vi "TMC module control_noVISA.vi"(8 "Winkel [°]":dbl min=-360.0 max=360.0 step=0.1, 9 "Nur Position auslesen":bool=TRUE, 10 "error in (no error)":errorcluster, 11 "VISA resource name":refnum<visa-resource-name>="COM6") -> (0 "Ausgelesener Winkel [°]":dbl format="%.1f", 1 "Fehler":bool, 2 "error out":errorcluster, 3 "VISA resource name out":refnum<visa-resource-name>)   [LabVIEW 2019]
doc: "Diese VI steuert einen Steppermotor mit TMCM-110 Modul.\nBei Start laufen folgende Schritte ab:\n1. Wenn \"nur Position auslesen\" deaktiviert ist\n- Überprüfe, ob neu gestartet wurde\n- falls ja: korregiere aktuelle Position auf letze Positionskoordinate vor Abschaltung\n- sende anzufahrende Position (Motor setzt sich in Bewegung)\n- Speichere neue Positions-Koordinate\n- lese aktuelle Position\n2. Wenn \"nur Position auslesen\" aktiviert\n- lese aktuelle Position\n\nDiese VI sollte nur ausgeführt werden, wenn vorher die VI \"Modul Reset\" auf den Motor\nausgeführt wurde"
panel:
  out "Schritte je Winkelgrad":dbl
  out "Auslgelesenes Array":u8[](array[numeric])
  out "Ausgegebener Wert\ndezimal":i32
  out "Type":string
  out "Data to write":string
  out "Instruction":string
  out "Motor":string
  out "Value":string
  # "Diese VI steuert einen Steppermotor mit TMCM-110 Modul.\nBei Start laufen folgende Schritte ab:\n1. Wenn \"nur Position auslesen\" deaktiviert ist\n- Überprüfe, ob neu gestartet wurde\n- falls ja: korregiere aktuelle Position auf letze Positionskoordinate vor Abschaltung\n- sende anzufahrende Position (Motor setzt sich in Bewegung)\n- Speichere neue Positions-Koordinate\n- lese aktuelle Position\n2. Wenn \"nur Position auslesen\" aktiviert\n- lese aktuelle Position\n\nDiese VI sollte nur ausgeführt werden, wenn vorher ein mal die VI \"Modul Reset\" auf den Motor\nausgeführt wurde"
  # "RS232 configuration"
  # "Winkel Eingabe und Auslese"
  # "Kontrolldaten"
  # "Leuchtet diese Lampe auf kann der Motor nicht ausgelesen werden!\nFolgende Ursachen sind möglich:\n-Motor hat keinen Strom\n-Motor ist nicht angeschlossen\n-RS232 Konfigurationen sind falsch"
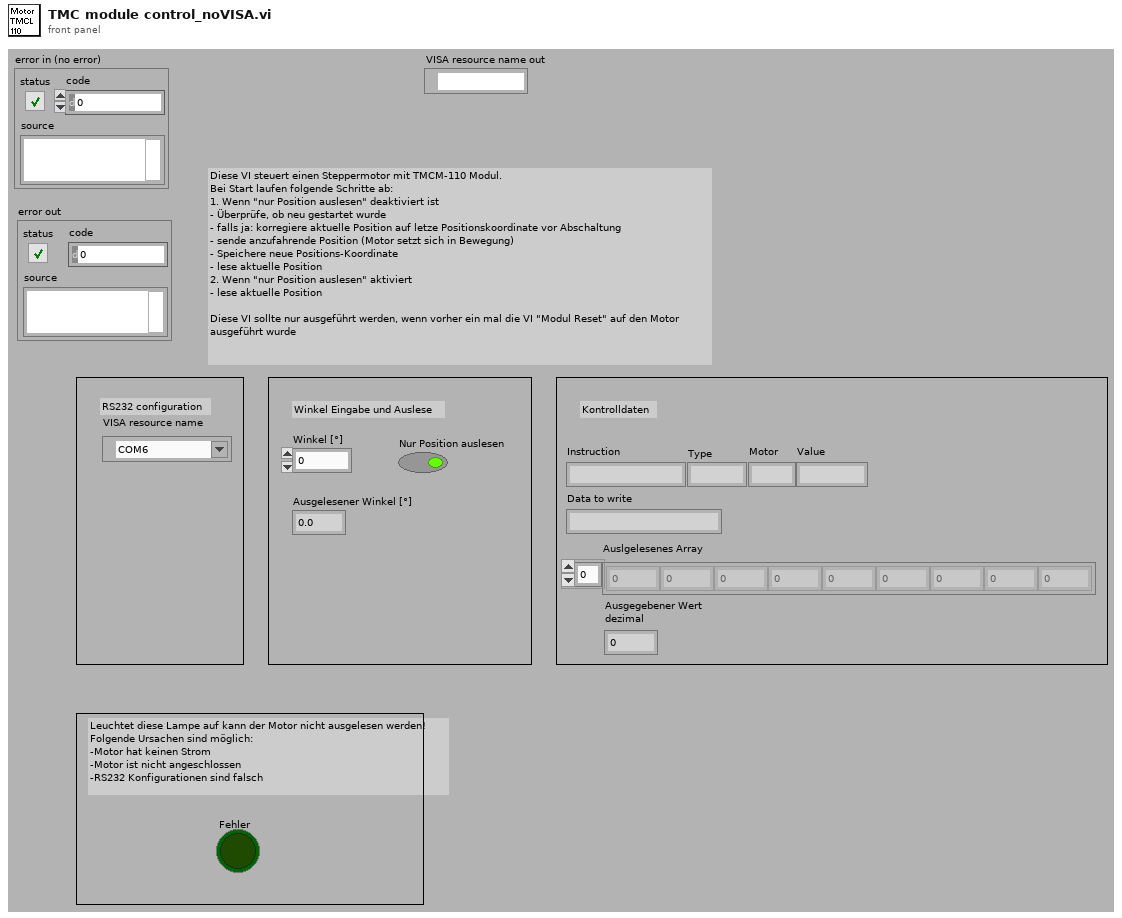
[diagram p1: front panel]
types:
  T1 = cluster{"Laufnummer":i32, "Aktuelle Position":i32, "Zielposition":i32, "gespeicherte Kooridnate":i32, "Case \"Neustart\"":bool}
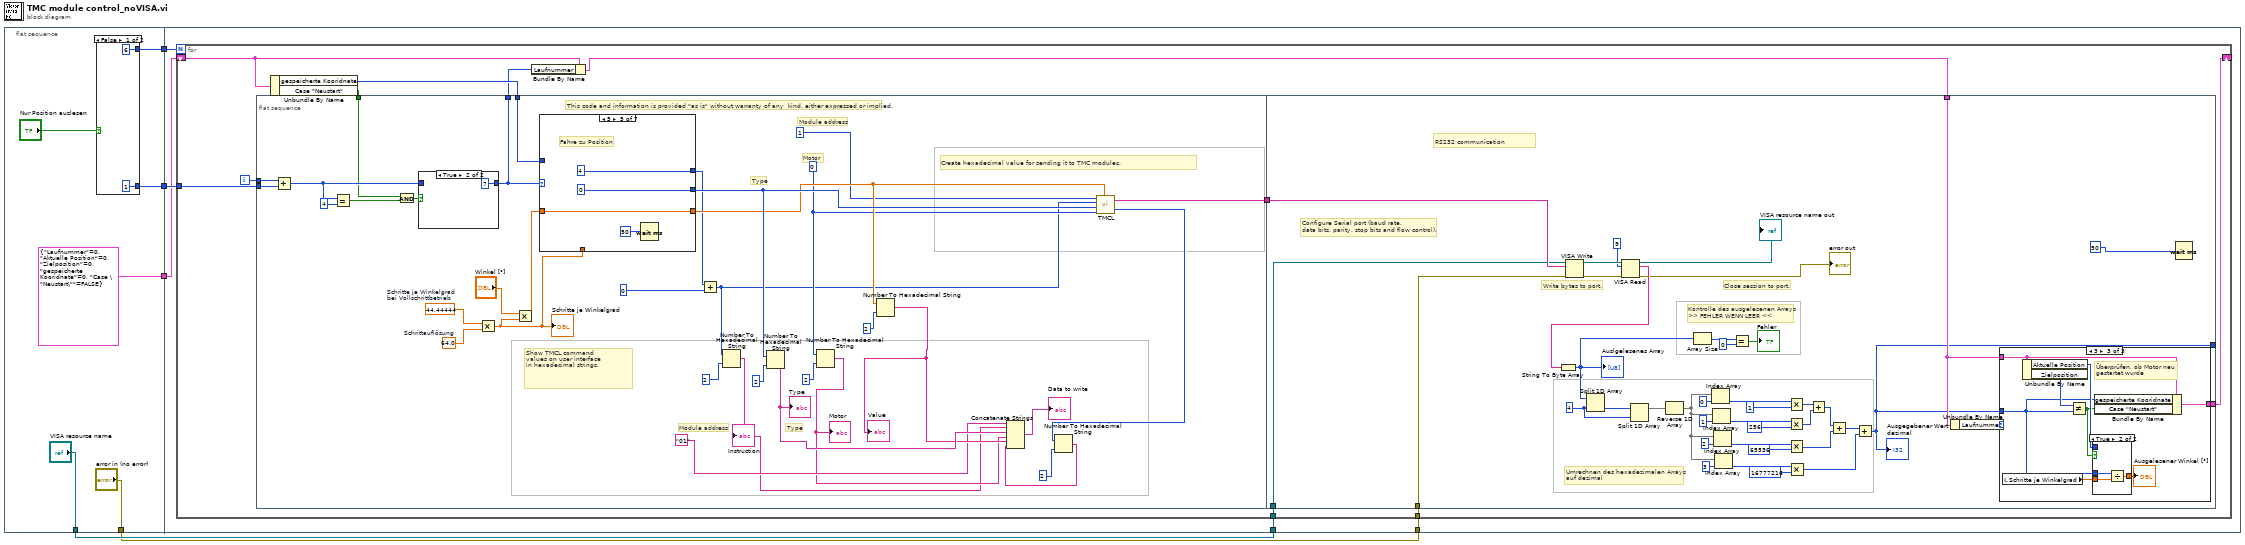
[diagram p0: block diagram]
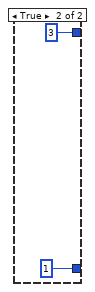
[diagram p2: hidden frame]
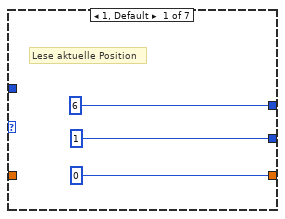
[diagram p4: hidden frame]
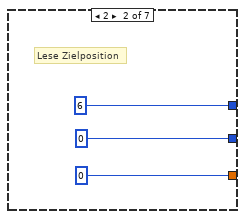
[diagram p5: hidden frame]
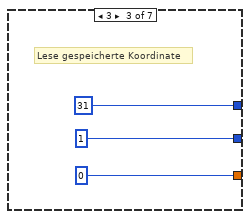
[diagram p6: hidden frame]
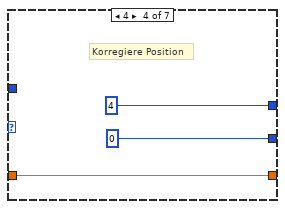
[diagram p7: hidden frame]
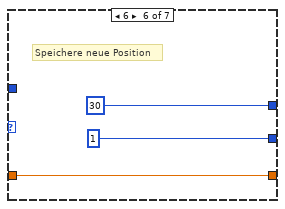
[diagram p8: hidden frame]
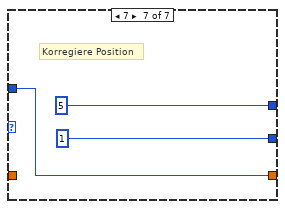
[diagram p9: hidden frame]
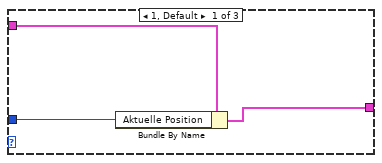
[diagram p10: hidden frame]
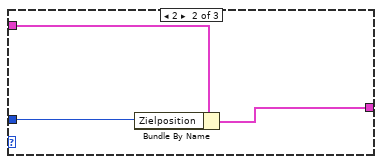
[diagram p11: hidden frame]
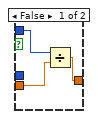
[diagram p12: hidden frame]
diagram:
  n1 = flat-sequence {
    tunnel: [w11] -> w5
    tunnel: [w9] -> w4
    tunnel: [T1 {"Laufnummer"=0, "Aktuelle Position"=0, "Zielposition"=0, "gespeicherte Kooridnate"=0, "Case \"Neustart\""=FALSE}] -> w3
    tunnel: ["VISA resource name"] -> w2
    tunnel: ["error in (no error)"] -> w1
    tunnel: w5 -> [w20]
    tunnel: w4 -> [w19]
    tunnel: w3 -> [w18]
    tunnel: w1 -> [w17]
    tunnel: w2 -> [w16]
    frame #0 {
      n2 = case shown="False" "Nur Position auslesen" {
        tunnel: [1 ("y") 1 ("y")] -> w11
        tunnel: [6 3] -> w9
        frame False {
        }
        frame True {
        }
      }
    }
    frame #1 {
      n3 = for {
        N: w19 -> [_]
        tunnel: w20 -> [w30]
        shift-right: [w28] -> _
        shift-left: w18 -> [w26]
        tunnel: w17 -> [w22]
        tunnel: w16 -> [w21]
        i -> [w31]
        n4 = flat-sequence {
          tunnel: w31 -> [w38]
          tunnel: [w46] -> w29
          tunnel: w30 -> [w44]
          tunnel: w27 -> [w40]
          tunnel: [w35] -> w24
          tunnel: w23 -> [w33]
          tunnel: [w100] -> _
          tunnel: w29 -> [w130]
          tunnel: w25 -> [w101]
          tunnel: [w99] -> w28
          tunnel: w22 -> [w94]
          tunnel: w21 -> [w93]
          frame #0 {
            w41 = 64.0  # Schrittauflösung
            w42 = 44.44444  # Schritte je Winkelgrad bei Vollschrittbetrieb
            w62 = 0 ("Motor")
            # "Motor"
            # "Type"
            # "This code and information is provided \"as is\" without warranty of any  kind, either expressed or implied."
            # "Create hexadecimal value for sending it to TMC modules."
            # "Show TMCL command\nvalues on user interface\nin hexadecimal strings."
            # "Type"
            # "Module address"
            # "Module address"
            n5 = Add(x=w38, y=w44) -> (x+y=w36:i32)
            n6 = Equal?(x=w36, y=4) -> (x = y?=w32:bool)
            n7 = And(x=w33, y=w32) -> (x .and. y?=w34:bool)
            n8 = case shown="True" w34 {
              tunnel: w36 -> [w67 _]
              tunnel: [w67 7] -> w35
              frame False {
              }
              frame True {
              }
            }
            n9 = Multiply(x=w42, y=w41) -> (x*y=w39:dbl)
            "Schritte je Winkelgrad" <- w39
            n10 = Multiply(x="Winkel [°]", y=w39) -> (x*y=w45:dbl)
            n11 = case shown="5" w35 {
              tunnel: [6 6 31 4 4 30 5] -> w61
              tunnel: [1 0 1 0 0 1 1] -> w65
              tunnel: [0 0 0 w78 w82 w85 w88] -> w63
              tunnel: w45 -> [_ _ _ w78 w82 w85 _]
              tunnel: w40 -> [_ _ _ _ _ _ w88]
              tunnel: w39 -> [_ _ _ _ _ _ _]
              frame 1, Default {
                # "Lese aktuelle Position"
              }
              frame 2 {
                # "Lese Zielposition"
              }
              frame 3 {
                # "Lese gespeicherte Koordinate"
              }
              frame 4 {
                # "Korregiere Position"
              }
              frame 5 {
                # "Fahre zu Position"
                n12 = Wait (ms)(milliseconds to wait=u32 50 ("Zu wartende ms")) -> ()  [unwired: 1 out]
              }
              frame 6 {
                # "Speichere neue Position"
              }
              frame 7 {
                # "Korregiere Position"
              }
            }
            n13 = Add(x=w61, y=0) -> (x+y=w56:i32)
            n14 = Number To Hexadecimal String(1:2, 2:w56) -> (0:w49:string)
            "Instruction" <- w49
            n15 = Number To Hexadecimal String(1:2, 2:w65) -> (0:w66:string)
            "Type" <- w66
            n16 = Number To Hexadecimal String(1:2, 2:w62) -> (0:w52:string)
            "Motor" <- w52
            n17 = Number To Hexadecimal String(1:2, 2:w63) -> (0:w59:string)
            "Value" <- w59
            n18 = call "TMCL.vi"("Address"=1, "Instruction"=w56, "Type"=w65, "Motor"=w62, "Value"=w63) -> ("Hexadecimal value"=w46:string, "CRC (Optional)"=w60:i32)
            n19 = Number To Hexadecimal String(1:2, 2:w60) -> (0:w55:string)
            n20 = Concatenate Strings("01", w49, w66, w52, w59, w55) -> (→"Data to write":string)
          }
          frame #1 {
            w123 = 4 ("Index")
            # "Umrechnen des hexadezimalen Arrays\nauf dezimal"
            # "Kontrolle des ausgelesenen Arrays\n>> FEHLER WENN LEER <<"
            # "RS232 communication"
            # "Write bytes to port."
            # "Configure Serial port (baud rate,\ndata bits, parity, stop bits and flow control)."
            # "Close session to port."
            n21 = VISA Write(VISA resource name=w93, write buffer=w130, error in (no error)=w94) -> (VISA resource name out=w127:refnum<visa-resource-name>, error out=w126:errorcluster)  [unwired: 1 out]
            n22 = VISA Read(VISA resource name=w127, byte count=u32 9 ("General Settings:Timeout Value"), error in (no error)=w126) -> (VISA resource name out=→"VISA resource name out":refnum<visa-resource-name>, read buffer=w129:string, error out=→"error out":errorcluster)  [unwired: 1 out]
            n23 = String To Byte Array(string=w129) -> (unsigned byte array=w98:u8[])
            "Auslgelesenes Array" <- w98
            n24 = Split 1D Array(array=w98, index=w123) -> (second subarray=w124:u8[])  [unwired: 1 out]
            n25 = Split 1D Array(array=w124, index=w123) -> (first subarray=w103:u8[])  [unwired: 1 out]
            n26 = Reverse 1D Array(array=w103) -> (reversed array=w117:u8[])
            n27 = Array Size(array=w98) -> (size(s)=w97:i32)
            n28 = Index Array(array=w117, index=0 ("Index")) -> (element=w113:u8)
            n29 = Index Array(array=w117, index=1 ("Index")) -> (element=w112:u8)
            n30 = Index Array(array=w117, index=2 ("Index")) -> (element=w111:u8)
            n31 = Index Array(array=w117, index=3 ("Index")) -> (element=w110:u8)
            n32 = Equal?(x=w97, y=0) -> (x = y?=→"Fehler":bool)
            n33 = Multiply(x=w113, y=1) -> (x*y=w109:i32)
            n34 = Multiply(x=w112, y=256) -> (x*y=w108:i32)
            n35 = Multiply(x=w111, y=65536) -> (x*y=w106:i32)
            n36 = Multiply(x=w110, y=16777216) -> (x*y=w105:i32)
            n37 = Add(x=w109, y=w108) -> (x+y=w107:i32)
            n38 = Add(x=w107, y=w106) -> (x+y=w104:i32)
            n39 = Add(x=w104, y=w105) -> (x+y=w100:i32)
            "Ausgegebener Wert\ndezimal" <- w100
            n40 = Unbundle By Name(w101) -> ("Laufnummer"=w102:i32)
            n41 = case shown="3" w102 {
              tunnel: w101 -> [w133 w136 w141]
              tunnel: [w132 w135 w140] -> w99
              tunnel: w100 -> [w131 w134 w138]
              frame 1, Default {
                n42 = Bundle By Name(cluster=w133, "Aktuelle Position"=w131) -> (w132:T1)
              }
              frame 2 {
                n43 = Bundle By Name(cluster=w136, "Zielposition"=w134) -> (w135:T1)
              }
              frame 3 {
                # "Überprüfen, ob Motor neu\ngestartet wurde"
                n44 = local read "Schritte je Winkelgrad"() -> (w144:dbl)
                n45 = Unbundle By Name(w141) -> ("Aktuelle Position"=w143:i32, "Zielposition"=w139:i32)
                n46 = Not Equal?(x=w139, y=w138) -> (x != y?=w137:bool)
                n47 = case shown="True" w137 {
                  tunnel: w143 -> [w147 _]
                  tunnel: w138 -> [_ w150]
                  tunnel: [w146 w149] -> w142
                  tunnel: w144 -> [w145 w148]
                  frame False {
                    n48 = Divide(x=w147, y=w145) -> (x/y=w146:dbl)
                  }
                  frame True {
                    n49 = Divide(x=w150, y=w148) -> (x/y=w149:dbl)
                  }
                }
                "Ausgelesener Winkel [°]" <- w142
                n50 = Bundle By Name(cluster=w141, "gespeicherte Kooridnate"=w138, "Case \"Neustart\""=w137) -> (w140:T1)
              }
            }
            n51 = Wait (ms)(milliseconds to wait=u32 50) -> ()  [unwired: 1 out]
          }
        }
        n52 = Unbundle By Name(w26) -> ("gespeicherte Kooridnate"=w27:i32, "Case \"Neustart\""=w23:bool)
        n53 = Bundle By Name(cluster=w26, "Laufnummer"=w24) -> (w25:T1)
      }
    }
  }
